vi "HTML_WriteDocToFile.vi"(8 "Error In":errorcluster, 9 ".html Filetext (In)":string, 10 "Savepath (.html)":path) -> (0 "Error Out":errorcluster, 2 "Savepath Dup (Out)":path)   [LabVIEW 2014]
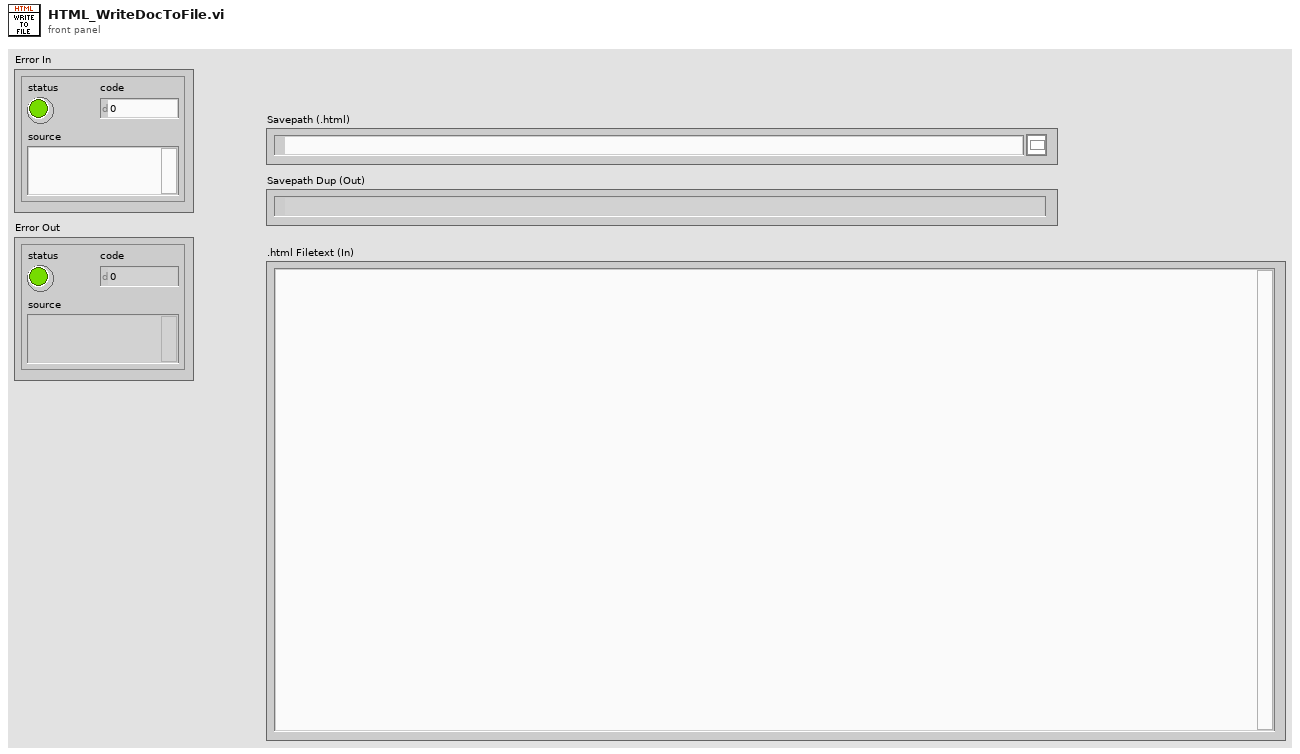
[diagram p1: front panel]
types:
  T1 = enum16{"open", "replace", "create", "open or create", "replace or create", "replace or create with confirmation"}
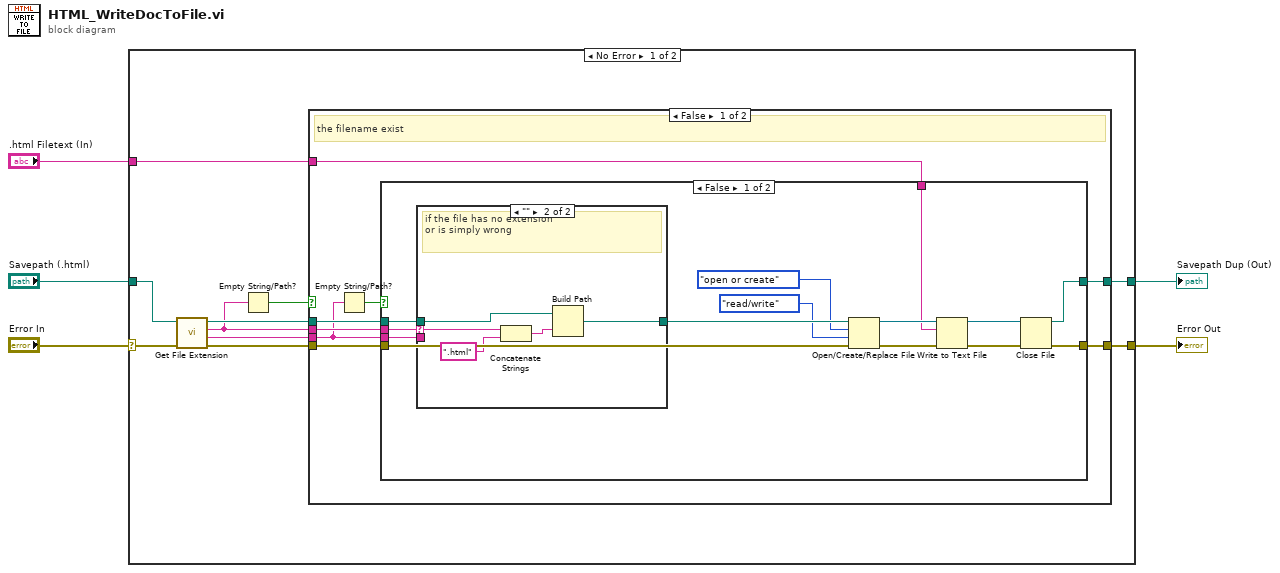
[diagram p0: block diagram]
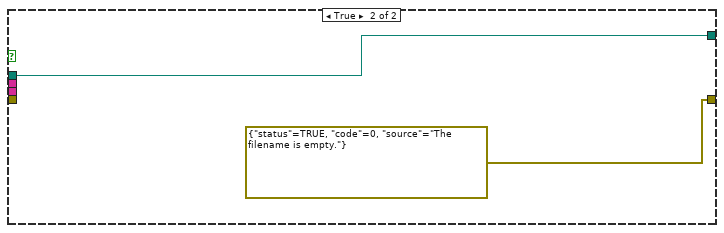
[diagram p3: hidden frame]
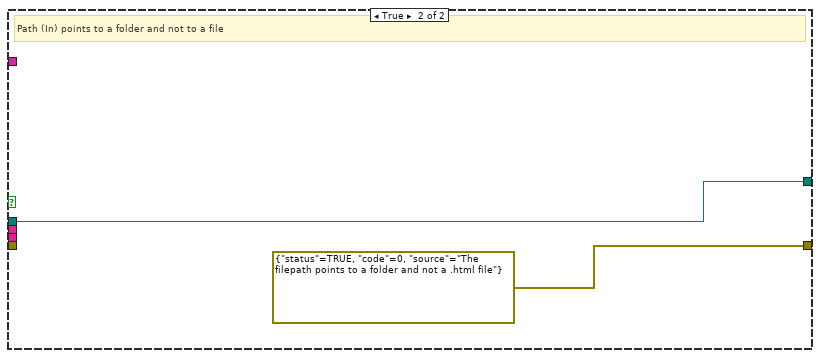
[diagram p4: hidden frame]
diagram:
  n1 = case shown="No Error" "Error In" {
    selector: "Error In" -> [w11 w49]
    tunnel: "Savepath (.html)" -> [w15 w48]
    tunnel: [w12 w49] -> w4
    tunnel: ".html Filetext (In)" -> [w10 _]
    tunnel: [w9 w48] -> w1
    frame No Error {
      n2 = call <vilib>:"Get File Extension.vi"("error in (no error)"=w11, "file"=w15) -> ("error out"=w13:errorcluster, "filename without extension"=w8:string, "lowercase file extension"=w6:string, "dup file"=w14:path)  [unwired: 5 in, 1 out]
      n3 = Empty String/Path?(string/path=w6) -> (empty?=w7:bool)
      n4 = case shown="False" w7 {
        tunnel: w6 -> [w23 _]
        tunnel: w8 -> [w17 _]
        tunnel: w14 -> [w22 w47]
        tunnel: w13 -> [w21 _]
        tunnel: [w20 errorcluster {"status"=TRUE, "code"=0, "source"="The filepath points to a folder and not a .html file"} ("error out")] -> w12
        tunnel: w10 -> [w19 _]
        tunnel: [w18 w47] -> w9
        frame False {
          # "the filename exist"
          n5 = Empty String/Path?(string/path=w17) -> (empty?=w16:bool)
          n6 = case shown="False" w16 {
            tunnel: w23 -> [w37 _]
            tunnel: w17 -> [w36 _]
            tunnel: w22 -> [w35 w44]
            tunnel: w21 -> [w33 _]
            tunnel: [w30 errorcluster {"status"=TRUE, "code"=0, "source"="The filename is empty."} ("error out")] -> w20
            tunnel: w19 -> [w25 _]
            tunnel: [w24 w44] -> w18
            frame False {
              n7 = case shown="\"\"" w37 {
                selector: w37 -> [_ w41]
                tunnel: w36 -> [_ _]
                tunnel: w35 -> [w38 w43]
                tunnel: [w38 w39] -> w34
                frame ".html", Default {
                }
                frame "" {
                  # "if the file has no extension\nor is simply wrong"
                  n8 = Concatenate Strings(w41, ".html" ("string")) -> (w42:string)
                  n9 = Build Path(base path=w43, name or relative path=w42) -> (appended path=w39:path)
                }
              }
              n10 = Open/Create/Replace File(file path (use dialog)=w34, error in=w33, operation (0:open)=T1."open or create", access (0:read/write)=enum16{"read/write", "read-only", "write-only"}."read/write") -> (refnum out=w27:refnum<file>, error out=w32:errorcluster)  [unwired: 2 in, 1 out]
              n11 = Write to Text File(file (use dialog)=w27, text=w25, error in=w32) -> (refnum out=w26:refnum<file>, error out=w31:errorcluster)  [unwired: 1 in, 1 out]
              n12 = Close File(refnum=w26, error in=w31) -> (path=w24:path, error out=w30:errorcluster)
            }
            frame True {
            }
          }
        }
        frame True {
          # "Path (In) points to a folder and not to a file"
        }
      }
    }
    frame Error {
    }
  }
  "Error Out" <- w4
  "Savepath Dup (Out)" <- w1
